vi "Enabled.vi"(7 "Label Text":string[](array[string]), 8 "error in (no error)":errorcluster, 11 "Ctl Refnum in":refnum<vi>) -> (0 "error out":errorcluster, 3 "Ctl Refnum out":refnum<vi>)   [LabVIEW 2017, in "Toolbox.lvlib"]
uses:
  Toolbox.lvlib
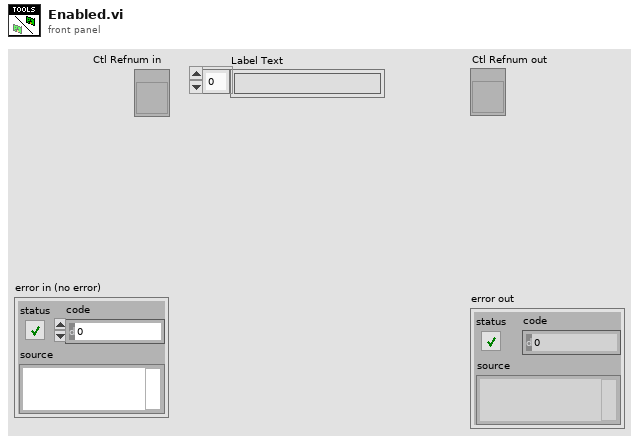
[diagram p1: front panel]
types:
  T1 = enum8{"Enabled", "Disabled", "Disabled and Grayed Out"}
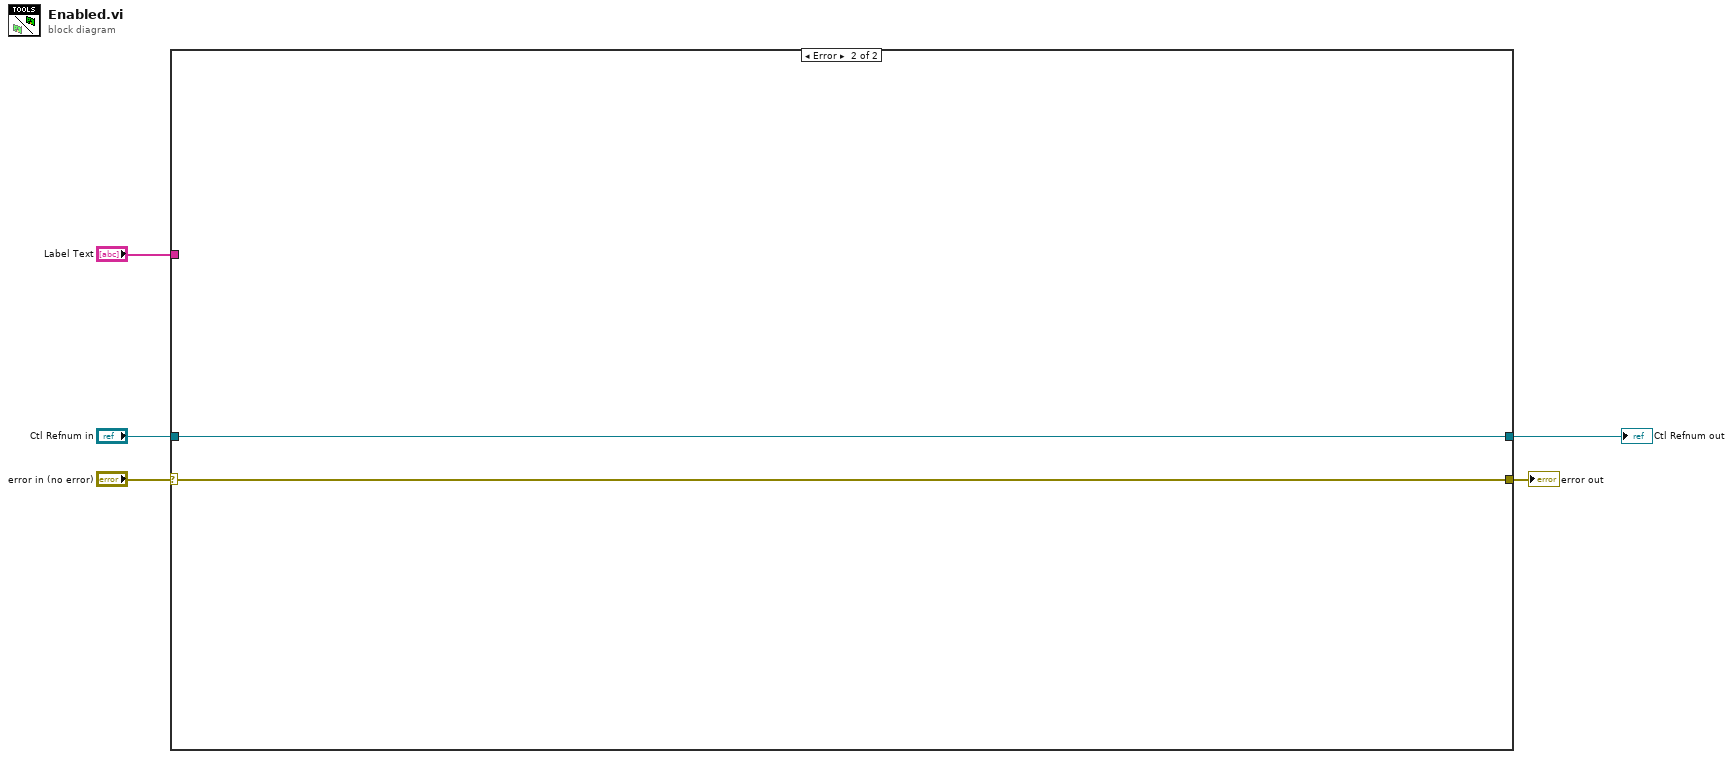
[diagram p0: block diagram]
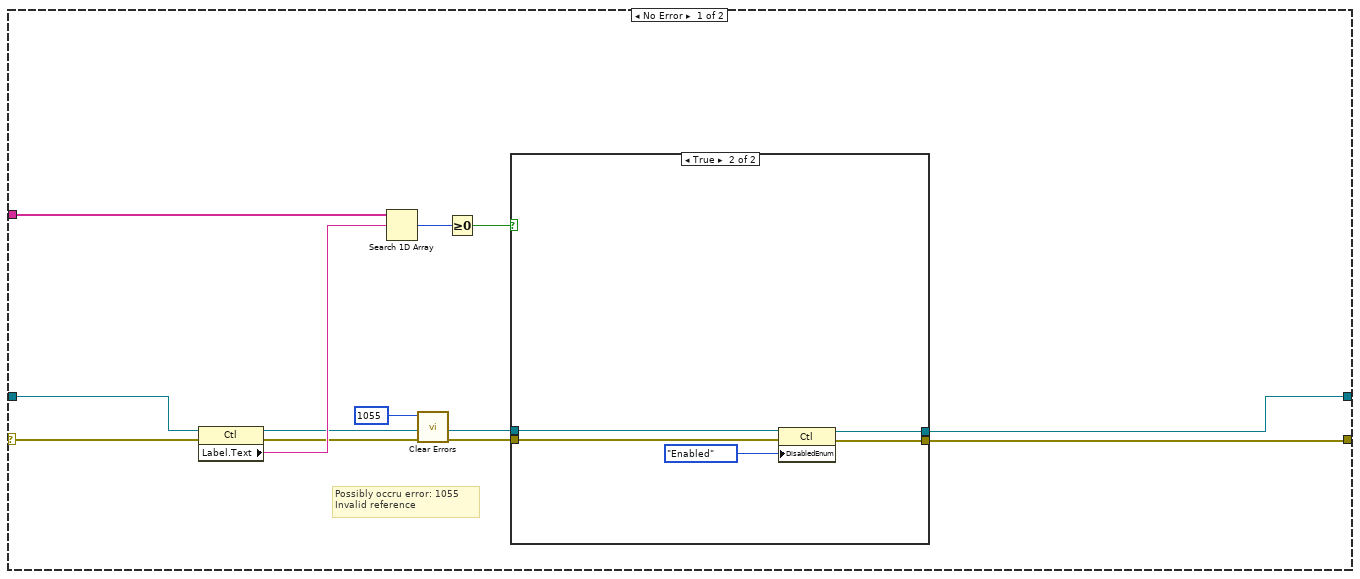
[diagram p2: hidden frame]
diagram:
  n1 = case shown="Error" "error in (no error)" {
    selector: "error in (no error)" -> [w17 w26]
    tunnel: [w9 w26] -> w4
    tunnel: "Ctl Refnum in" -> [w16 w25]
    tunnel: "Label Text" -> [w15 _]
    tunnel: [w6 w25] -> w1
    frame No Error {
      # "Possibly occru error: 1055\nInvalid reference"
      n2 = property class="Ctl"(reference=w16, error in=w17) -> (reference out=w12:refnum<vi>, error out=w13:errorcluster, "Label.Text"=w14:string)
      n3 = Search 1D Array(1D array=w15, element=w14) -> (index of element=w11:i32)  [unwired: 1 in]
      n4 = call <vilib>:"Clear Errors.vi"("error in (no error)"=w13, "specific error code to clear (0: all)"=1055) -> ("error out"=w8:errorcluster)  [unwired: 4 in, 1 out]
      n5 = Greater Or Equal To 0?(x=w11) -> (x >= 0?=w10:bool)
      n6 = case shown="True" w10 {
        tunnel: w8 -> [w19 w24]
        tunnel: w12 -> [w18 w23]
        tunnel: [w19 w21] -> w9
        tunnel: [w18 w20] -> w6
        frame False {
        }
        frame True {
          n7 = property class="Ctl"(reference=w23, error in=w24, "DisabledEnum"=T1."Enabled" ("Disabled")) -> (reference out=w20:refnum<vi>, error out=w21:errorcluster)
        }
      }
    }
    frame Error {
    }
  }
  "error out" <- w4
  "Ctl Refnum out" <- w1
